vi "Get_AppINI_GenericSettings.vi"(8 "error in (no error)":errorcluster, 11 "EVE in":refnum<class "EVE.lvclass">) -> (0 "error out":errorcluster, 3 "EVE out":refnum<class "EVE.lvclass">)   [LabVIEW 2013, in "EVE.lvclass"]
uses:
  EVE.lvclass
  EVE.lvclass/EVE.ctl
  App_GenericSettings.ctl
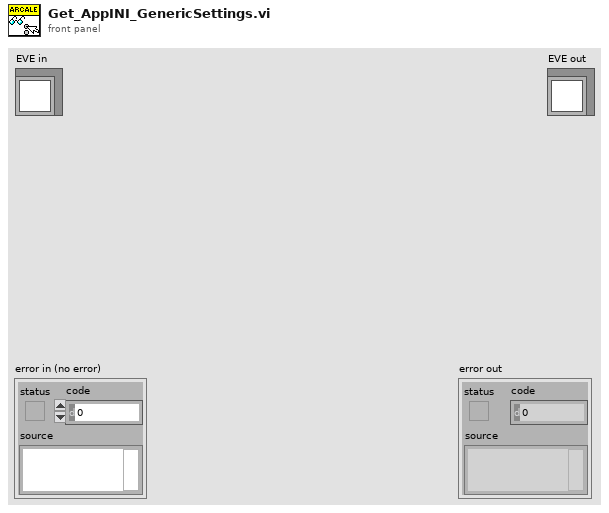
[diagram p1: front panel]
types:
  T1 = typedef "EVE.lvclass/App_GenericSettings.ctl" = cluster{"SpecificSettings":cluster{"FolderPath":path, "XMLFile":string}, "Log":cluster{"MaxLogFiles":i32, "MaxLogMessagesPerFile":i32}, "Debug":cluster{"Active":bool}, "Dictionnary":cluster{"FolderPath":path, "TradFile":string}, "Ressources":cluster{"FolderPath":path}}
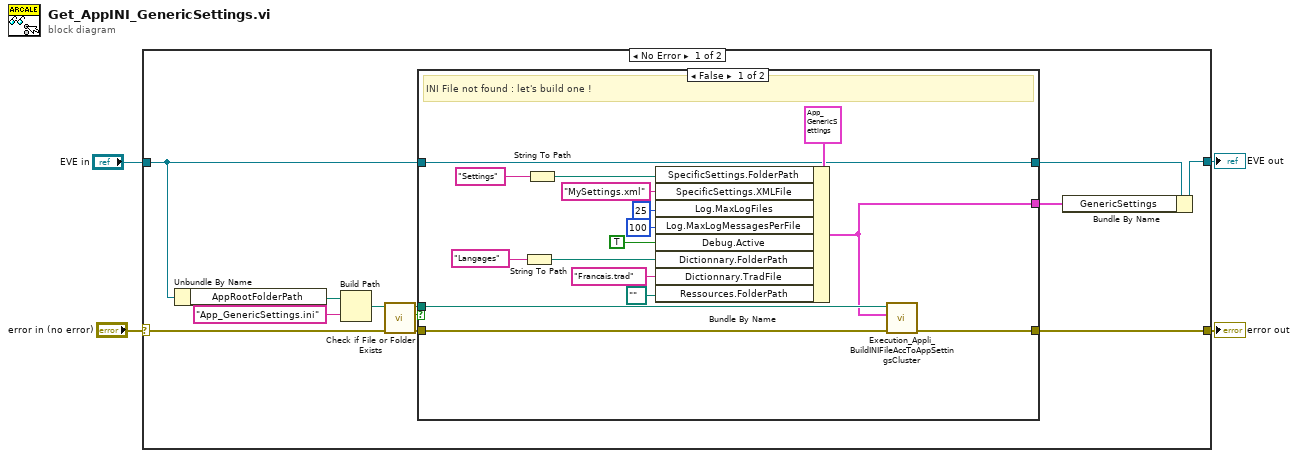
[diagram p0: block diagram]
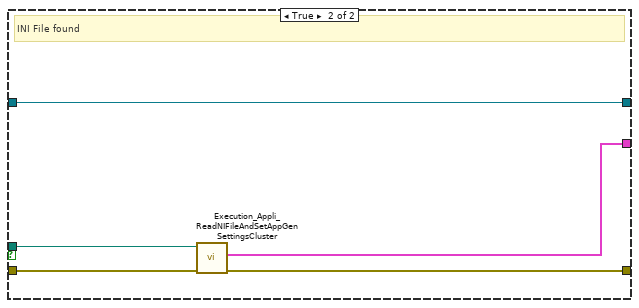
[diagram p2: hidden frame]
diagram:
  n1 = case shown="No Error" "error in (no error)" {
    selector: "error in (no error)" -> [w14 w39]
    tunnel: [w5 w39] -> w3
    tunnel: [w9 w38] -> w1
    tunnel: "EVE in" -> [w7 w38]
    frame No Error {
      n2 = Unbundle By Name(w7) -> ("AppRootFolderPath"=w10:path)
      n3 = Build Path(base path=w10, name or relative path="App_GenericSettings.ini") -> (appended path=w15:path)
      n4 = call <vilib>:"Check if File or Folder Exists.vi"("error in (no error)"=w14, "path"=w15) -> ("error out"=w11:errorcluster, "file or folder exists?"=w13:bool, "dup path"=w12:path)  [unwired: 7 in]
      n5 = case shown="False" w13 {
        tunnel: w12 -> [w24 w37]
        tunnel: w11 -> [w26 w36]
        tunnel: [w23 w33] -> w8
        tunnel: w7 -> [w25 w34]
        tunnel: [w25 w34] -> w6
        tunnel: [w22 w35] -> w5
        frame False {
          # "INI File not found : let's build one !"
          n6 = String To Path(string="Langages" ("name or relative path")) -> (path=w17:path)
          n7 = String To Path(string="Settings" ("name or relative path")) -> (path=w19:path)
          n8 = Bundle By Name(cluster=T1 {"SpecificSettings"={"FolderPath"=path "", "XMLFile"=""}, "Log"={"MaxLogFiles"=0, "MaxLogMessagesPerFile"=0}, "Debug"={"Active"=FALSE}, "Dictionnary"={"FolderPath"=path "", "TradFile"=""}, "Ressources"={"FolderPath"=path ""}} ("GenericSettings"), "SpecificSettings.FolderPath"=w19, "SpecificSettings.XMLFile"="MySettings.xml", "Log.MaxLogFiles"=25, "Log.MaxLogMessagesPerFile"=100, "Debug.Active"=TRUE, "Dictionnary.FolderPath"=w17, "Dictionnary.TradFile"="Francais.trad", "Ressources.FolderPath"=path "") -> (w23:T1)
          n9 = call "Execution_Appli_BuildINIFileAccToAppSettingsCluster.vi"("error in"=w26, "GenericSettings"=w23, "INI Path"=w24) -> ("error out"=w22:errorcluster)  [unwired: 8 in]
        }
        frame True {
          # "INI File found"
          n10 = call "Execution_Appli_ReadNIFileAndSetAppGenSettingsCluster.vi"("error in"=w36, "INI Path"=w37) -> ("error out"=w35:errorcluster, "GenericSettings"=w33:T1)  [unwired: 8 in]
        }
      }
      n11 = Bundle By Name(cluster=w6, "GenericSettings"=w8) -> (w9:refnum<class "EVE.lvclass">)
    }
    frame Error {
    }
  }
  "error out" <- w3
  "EVE out" <- w1
